vi "Periodic Tasks.vi"(8 "error in":errorcluster) -> ()   [LabVIEW 2013]
doc: "This VI runs in parallel to other tasks. It can contain as many user-defined periodic loops as you need. These can carry out PID or other sorts of timed response."
uses:
  <vilib>/Rock Robotics/SystemInterfaces/Utilities/FPGA_UtilitiesLED Source.ctl
  <vilib>/Rock Robotics/SystemInterfaces/Utilities/FPGA_UtilitiesLED State.ctl
  <vilib>/Rock Robotics/WPI/DriverStation/DriverStationLCD/WPI_DriverStationLCDLCDLine.ctl
  Robot Global Data.vi
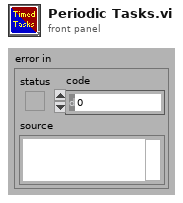
[diagram p1: front panel]
types:
  T1 = typedef "WPI_DigitalInputDevRef.ctl" = cluster{"DevStatus":errorcluster, "DIO Channel":T2, "Digital Module":T3}
  T2 = typedef "FPGA_DIOChannel.ctl" = enum8{"DIO 1", "DIO 2", "DIO 3", "DIO 4", "DIO 5", "DIO 6", "DIO 7", "DIO 8", "DIO 9", "DIO 10", "DIO 11", "DIO 12", "DIO 13", "DIO 14", "Invalid"}
  T3 = typedef "FPGA_TypedefDigitalModule.ctl" = enum16{"Digital Module 1", "Digital Module 2"}
  T4 = typedef "WPI_AnalogChannelDevRef.ctl" = cluster{"DevStatus":errorcluster, "Analog Module":T5, "Analog Channel":T6}
  T5 = typedef "FPGA_TypedefAnalogModule.ctl" = enum16{"Analog Module 1", "Analog Module 2"}
  T6 = typedef "FPGA_AIChannel.ctl" = enum8{"AI 1", "AI 2", "AI 3", "AI 4", "AI 5", "AI 6", "AI 7", "AI 8", "Invalid"}
  T7 = typedef "WPI_EncoderDevRef.ctl" = cluster{"DevStatus":errorcluster, "EncoderIndex":T8, "CounterIndex":T9, "DistancePerCount":dbl, "Decoding Type":T10}
  T8 = typedef "FPGA_EncoderIdx.ctl" = enum8{"Enc 0", "Enc 1", "Enc 2", "Enc 3", "Invalid"}
  T9 = typedef "FPGA_CounterCtrSystemIndex.ctl" = enum8{"Ctr 0", "Ctr 1", "Ctr 2", "Ctr 3", "Ctr 4", "Ctr 5", "Ctr 6", "Ctr 7", "Invalid"}
  T10 = typedef "WPI_EncoderType.ctl" = enum16{"1x", "2x", "4x"}
  T11 = cluster{"Winch Desired Location":dbl, "Winch Desired Location 2":dbl, "Winch Desired Location 3":dbl}
  T12 = typedef "FPGA_UtilitiesLED State.ctl" = enum16{"Off", "On", "Toggle"}
  T13 = typedef "FPGA_UtilitiesLED Source.ctl" = enum16{"User LED", "FPGA LED"}
  T14 = typedef "WPI_DriverStationLCDLCDLine.ctl" = enum16{"Main - Line 1", "User - Line 2", "User - Line 3", "User - Line 4", "User - Line 5", "User - Line 6"}
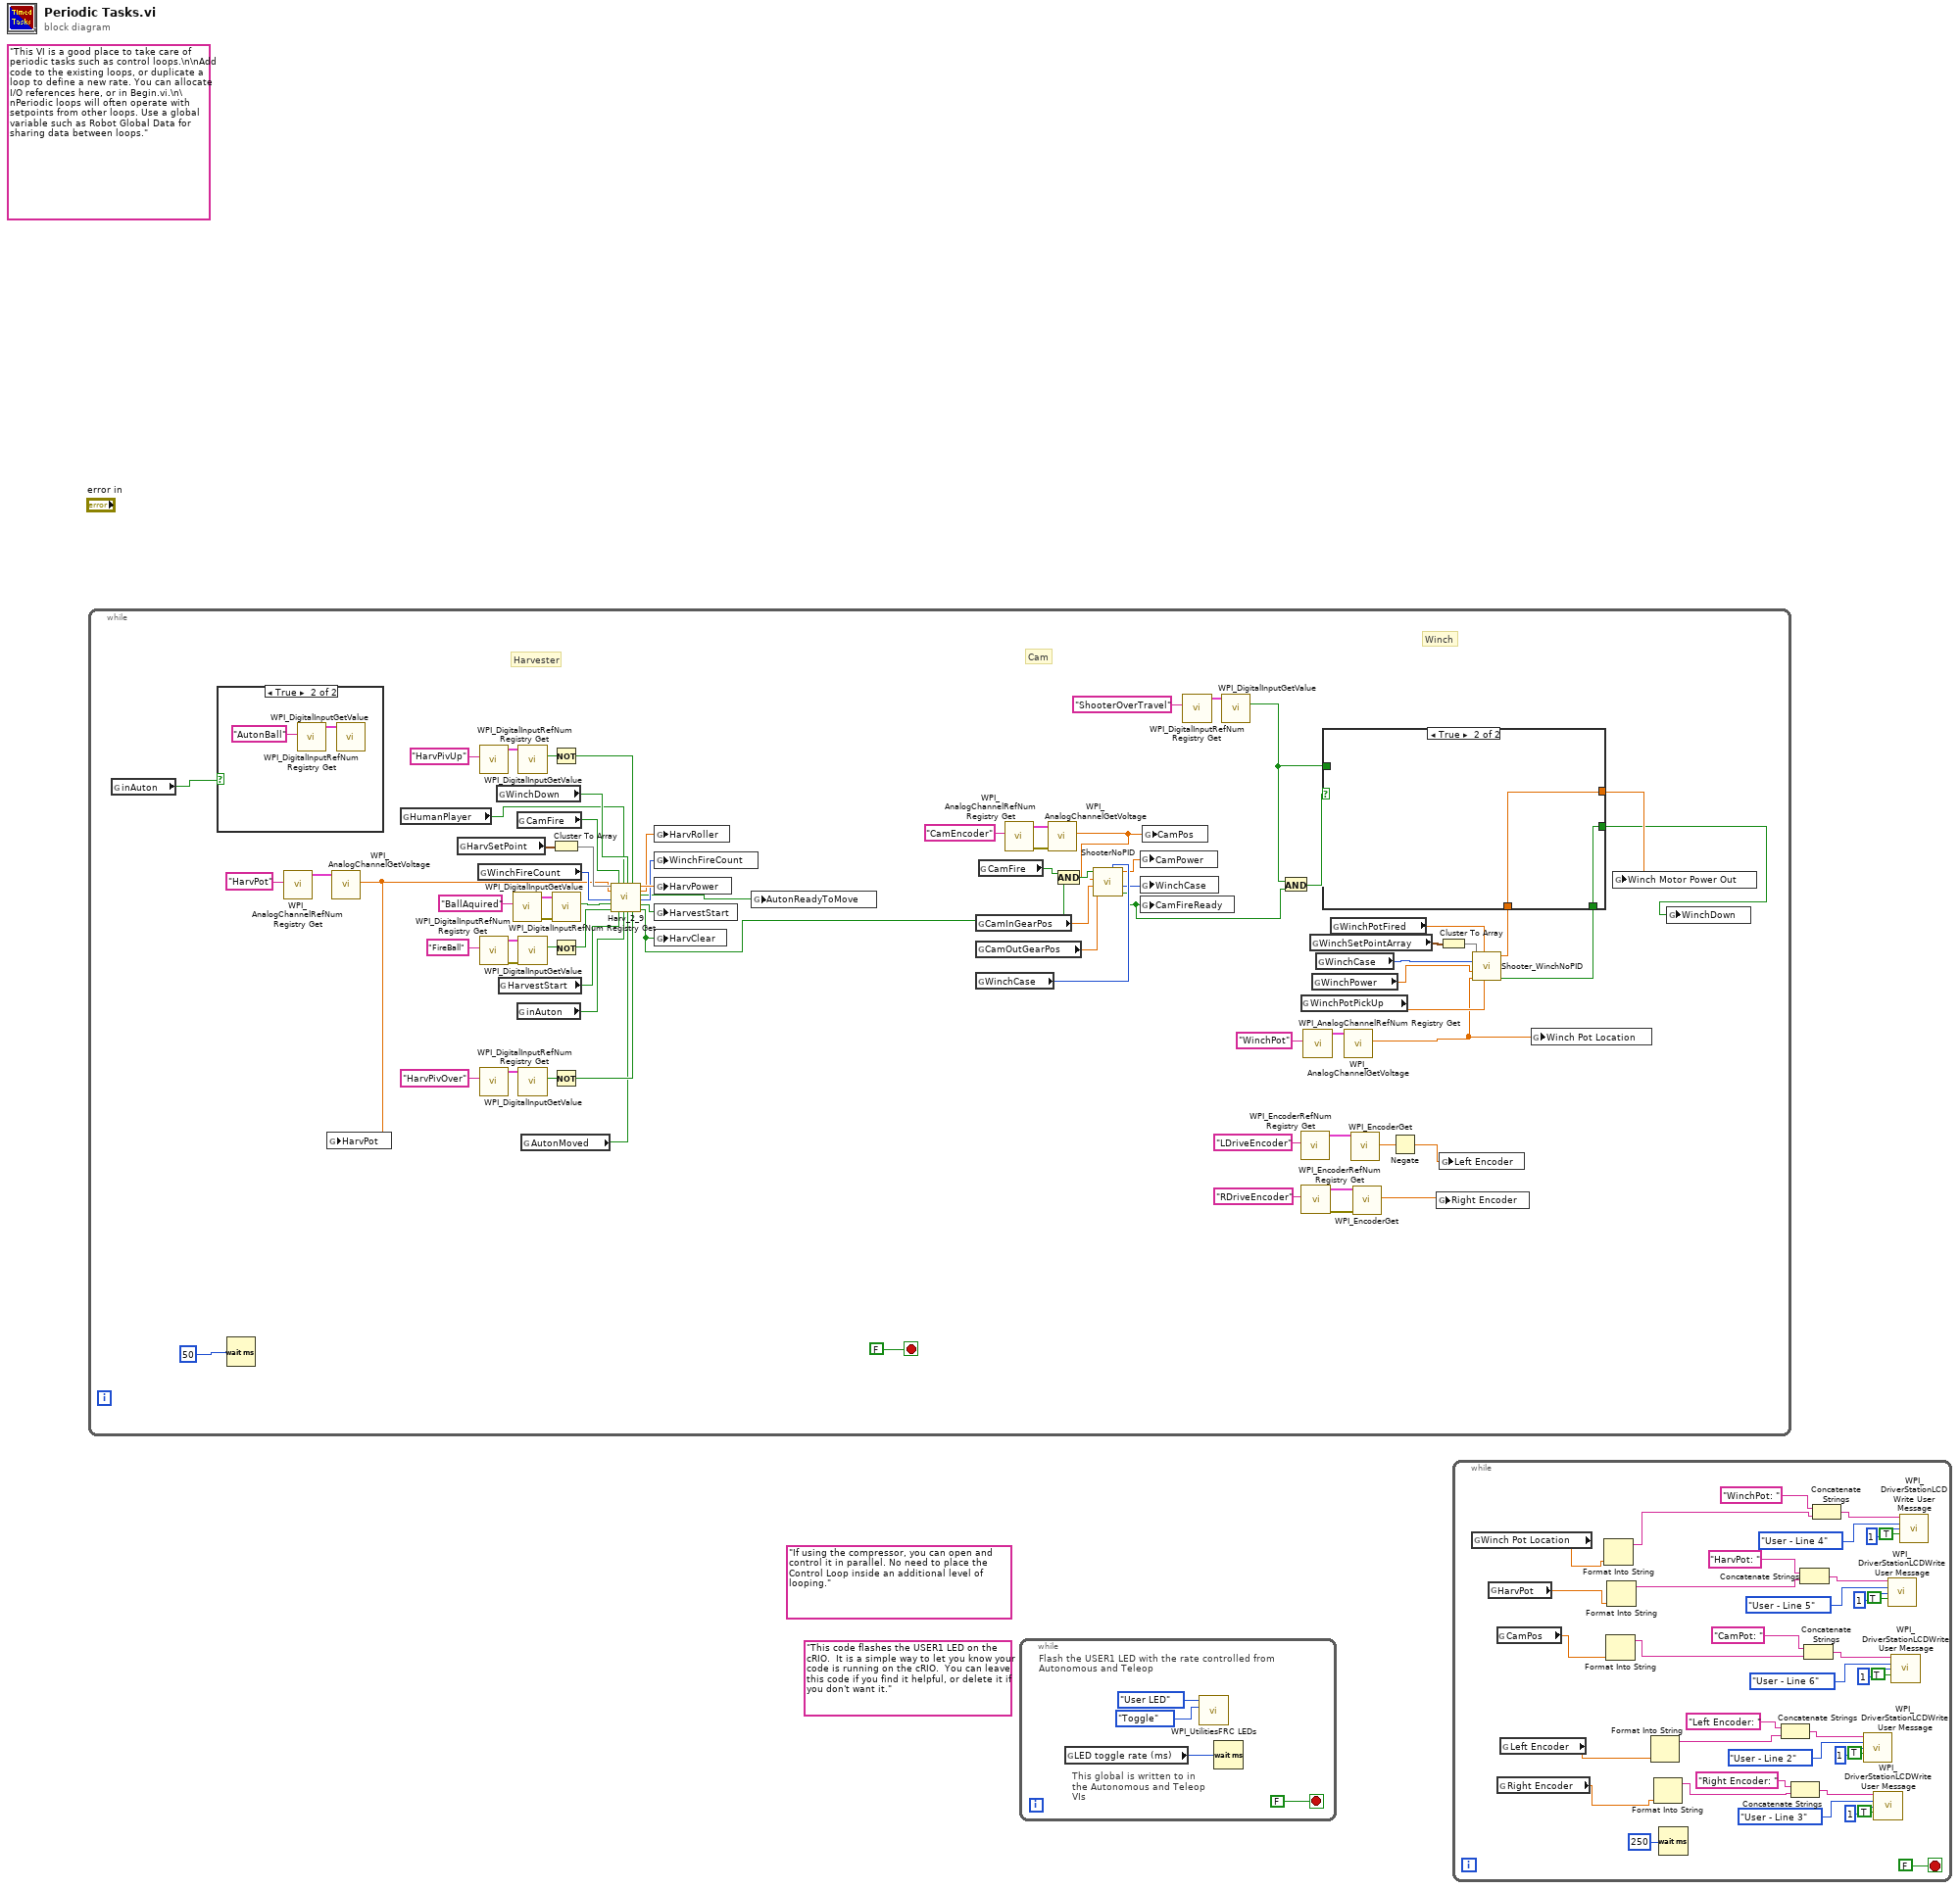
[diagram p0: block diagram]
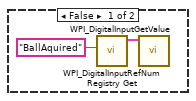
[diagram p2: hidden frame]
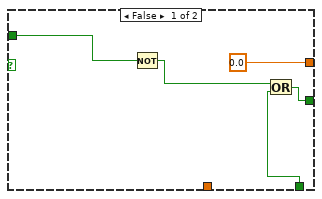
[diagram p3: hidden frame]
diagram:
  (unwired) "If using the compressor, you can open and control it in parallel. No need to place the Control Loop inside an additional level of looping."
  (unwired) "This code flashes the USER1 LED on the cRIO.  It is a simple way to let you know your code is running on the cRIO.  You can leave this code if you find it helpful, or delete it if you don't want it."
  (unwired) "This VI is a good place to take care of periodic tasks such as control loops.\n\nAdd code to the existing loops, or duplicate a loop to define a new rate. You can allocate I/O references here, or in Begin.vi.\n\nPeriodic loops will often operate with setpoints from other loops. Use a global variable such as Robot Global Data for sharing data between loops."
  n1 = while {
    stop <- FALSE stop-if-true
    # "Winch"
    # "Cam"
    # "Harvester"
    n2 = global read "Robot Global Data.vi" "inAuton"() -> (w1:bool)
    n3 = case shown="True" w1 {
      frame False {
        n4 = call <vilib>:"WPI_DigitalInputRefNum Registry Get.vi"("refnum name"="BallAquired") -> ("DigitalInputDevRef"=w77:T1)  [unwired: 9 in, 1 out]
        n5 = call <vilib>:"WPI_DigitalInputGetValue.vi"("DigitalInputDevRef"=w77) -> ()  [unwired: 8 in, 3 out]
      }
      frame True {
        n6 = call <vilib>:"WPI_DigitalInputRefNum Registry Get.vi"("refnum name"="AutonBall") -> ("DigitalInputDevRef"=w79:T1)  [unwired: 9 in, 1 out]
        n7 = call <vilib>:"WPI_DigitalInputGetValue.vi"("DigitalInputDevRef"=w79) -> ()  [unwired: 8 in, 3 out]
      }
    }
    n8 = Wait (ms)(milliseconds to wait=u32 50) -> ()  [unwired: 1 out]
    n9 = call <vilib>:"WPI_AnalogChannelRefNum Registry Get.vi"("refnum name"="HarvPot") -> ("AIDeviceRef"=w74:T4)  [unwired: 9 in, 1 out]
    n10 = call <vilib>:"WPI_AnalogChannelGetVoltage.vi"("AIDeviceRef"=w74) -> ("Voltage"=w13:dbl)  [unwired: 8 in, 2 out]
    n11 = global write "Robot Global Data.vi" "HarvPot"(w13) -> ()
    n12 = global read "Robot Global Data.vi" "HumanPlayer"() -> (w4:bool)
    n13 = global read "Robot Global Data.vi" "HarvSetPoint"() -> (w41:cluster{"Out":dbl, "In":dbl, "Clear":dbl})
    n14 = global read "Robot Global Data.vi" "WinchFireCount"() -> (w16:i32)
    n15 = call <vilib>:"WPI_DigitalInputRefNum Registry Get.vi"("refnum name"="HarvPivUp") -> ("DigitalInputDevRef"=w58:T1)  [unwired: 9 in, 1 out]
    n16 = call <vilib>:"WPI_DigitalInputRefNum Registry Get.vi"("refnum name"="FireBall") -> ("error out"=w47:errorcluster, "DigitalInputDevRef"=w48:T1)  [unwired: 9 in]
    n17 = call <vilib>:"WPI_DigitalInputRefNum Registry Get.vi"("refnum name"="HarvPivOver") -> ("DigitalInputDevRef"=w66:T1)  [unwired: 9 in, 1 out]
    n18 = global read "Robot Global Data.vi" "WinchDown"() -> (w34:bool)
    n19 = global read "Robot Global Data.vi" "HarvestStart"() -> (w45:bool)
    n20 = call <vilib>:"WPI_DigitalInputRefNum Registry Get.vi"("refnum name"="BallAquired") -> ("error out"=w54:errorcluster, "DigitalInputDevRef"=w53:T1)  [unwired: 9 in]
    n21 = global read "Robot Global Data.vi" "CamFire"() -> (w46:bool)
    n22 = global read "Robot Global Data.vi" "inAuton"() -> (w18:bool)
    n23 = call <vilib>:"WPI_DigitalInputGetValue.vi"("DigitalInputDevRef"=w58) -> ("Value"=w37:bool)  [unwired: 8 in, 2 out]
    n24 = call <vilib>:"WPI_DigitalInputGetValue.vi"("error in (no error)"=w47, "DigitalInputDevRef"=w48) -> ("Value"=w44:bool)  [unwired: 7 in, 2 out]
    n25 = call <vilib>:"WPI_DigitalInputGetValue.vi"("DigitalInputDevRef"=w66) -> ("Value"=w39:bool)  [unwired: 8 in, 2 out]
    n26 = global read "Robot Global Data.vi" "AutonMoved"() -> (w3:bool)
    n27 = Not(x=w37) -> (.not. x?=w36:bool)
    n28 = Cluster To Array(cluster=w41) -> (array=w40:dbl[])
    n29 = call <vilib>:"WPI_DigitalInputGetValue.vi"("error in (no error)"=w54, "DigitalInputDevRef"=w53) -> ("Value"=w43:bool)  [unwired: 7 in, 2 out]
    n30 = Not(x=w44) -> (.not. x?=w42:bool)
    n31 = Not(x=w39) -> (.not. x?=w38:bool)
    n32 = call "Harv_2_9.vi"("HarvSetpoints"=w40, "HarvPot"=w13, "Count"=w16, "BallAcquired"=w43, "FireBallSen"=w42, "Fire"=w46, "Harvest"=w45, "HPButton"=w4, "inAuton?"=w18, "WinchDown"=w34, "AutonMoved"=w3, "HarvPivUP"=w36, "HarvPivPickupLim"=w38) -> ("HarvPower"=w51:dbl, "HarvRoller"=w50:dbl, "AutonReadyToMove"=w2:bool, "CountOut"=w15:i32, "HarvStart"=w35:bool, "HarvCleared"=w8:bool)  [unwired: 1 in]
    n33 = global write "Robot Global Data.vi" "HarvRoller"(w50) -> ()
    n34 = global write "Robot Global Data.vi" "WinchFireCount"(w15) -> ()
    n35 = global write "Robot Global Data.vi" "HarvPower"(w51) -> ()
    n36 = global write "Robot Global Data.vi" "HarvestStart"(w35) -> ()
    n37 = global write "Robot Global Data.vi" "HarvClear"(w8) -> ()
    n38 = global write "Robot Global Data.vi" "AutonReadyToMove"(w2) -> ()
    n39 = global read "Robot Global Data.vi" "CamInGearPos"() -> (w23:dbl)
    n40 = global read "Robot Global Data.vi" "CamOutGearPos"() -> (w22:dbl)
    n41 = global read "Robot Global Data.vi" "WinchCase"() -> (w24:i32)
    n42 = global read "Robot Global Data.vi" "CamFire"() -> (w60:bool)
    n43 = call <vilib>:"WPI_AnalogChannelRefNum Registry Get.vi"("refnum name"="CamEncoder") -> ("error out"=w62:errorcluster, "AIDeviceRef"=w61:T4)  [unwired: 9 in]
    n44 = call <vilib>:"WPI_AnalogChannelGetVoltage.vi"("error in (no error)"=w62, "AIDeviceRef"=w61) -> ("Voltage"=w12:dbl)  [unwired: 7 in, 2 out]
    n45 = And(x=w60, y=w8) -> (x .and. y?=w25:bool)
    n46 = call "ShooterNoPID.vi"("WinchCaseIn"=w24, "InGearPosLow"=w22, "InGearPosHigh"=w23, "Pot"=w12, "Fire"=w25) -> ("There?"=w19:bool, "WinchCase"=w20:i32, "Power"=w21:dbl)  [unwired: 4 in]
    n47 = global write "Robot Global Data.vi" "CamPower"(w21) -> ()
    n48 = global write "Robot Global Data.vi" "WinchCase"(w20) -> ()
    n49 = global write "Robot Global Data.vi" "CamFireReady"(w19) -> ()
    n50 = global write "Robot Global Data.vi" "CamPos"(w12) -> ()
    n51 = call <vilib>:"WPI_DigitalInputRefNum Registry Get.vi"("refnum name"="ShooterOverTravel") -> ("DigitalInputDevRef"=w57:T1)  [unwired: 9 in, 1 out]
    n52 = call <vilib>:"WPI_DigitalInputGetValue.vi"("DigitalInputDevRef"=w57) -> ("Value"=w33:bool)  [unwired: 8 in, 2 out]
    n53 = And(x=w33, y=w19) -> (x .and. y?=w55:bool)
    n54 = global read "Robot Global Data.vi" "WinchPotPickUp"() -> (w17:dbl)
    n55 = call <vilib>:"WPI_EncoderRefNum Registry Get.vi"("refnum name"="LDriveEncoder") -> ("EncoderDevRef"=w68:T7)  [unwired: 9 in, 1 out]
    n56 = call <vilib>:"WPI_EncoderRefNum Registry Get.vi"("refnum name"="RDriveEncoder") -> ("error out"=w11:errorcluster, "EncoderDevRef"=w10:T7)  [unwired: 9 in]
    n57 = call <vilib>:"WPI_AnalogChannelRefNum Registry Get.vi"("refnum name"="WinchPot") -> ("AIDeviceRef"=w70:T4)  [unwired: 9 in, 1 out]
    n58 = global read "Robot Global Data.vi" "WinchSetPointArray"() -> (w30:T11)
    n59 = global read "Robot Global Data.vi" "WinchPower"() -> (w32:dbl)
    n60 = global read "Robot Global Data.vi" "WinchCase"() -> (w29:i32)
    n61 = global read "Robot Global Data.vi" "WinchPotFired"() -> (w5:dbl)
    n62 = call <vilib>:"WPI_AnalogChannelGetVoltage.vi"("AIDeviceRef"=w70) -> ("Voltage"=w14:dbl)  [unwired: 8 in, 2 out]
    n63 = call <vilib>:"WPI_EncoderGet.vi"("EncoderDevRef"=w68) -> ("Distance"=w7:dbl)  [unwired: 5 in, 5 out]
    n64 = call <vilib>:"WPI_EncoderGet.vi"("error in (no error)"=w11, "EncoderDevRef"=w10) -> ("Distance"=w9:dbl)  [unwired: 4 in, 5 out]
    n65 = Negate(x=w7) -> (-x=w6:dbl)
    n66 = global write "Robot Global Data.vi" "Right Encoder"(w9) -> ()
    n67 = Cluster To Array(cluster=w30) -> (array=w31:dbl[])
    n68 = global write "Robot Global Data.vi" "Left Encoder"(w6) -> ()
    n69 = call "Shooter_WinchNoPID.vi"("PickStartPos"=w17, "WinchFiredPos"=w5, "Winch Pot Location"=w14, "WinchPower"=w32, "selectedCase"=w29, "SetPointArray"=w31) -> ("isThere?"=w27:bool, "Winch Motor Power Out"=w26:dbl)  [unwired: 4 in]
    n70 = case shown="True" w55 {
      tunnel: [0.0 ("Winch Motor Power Out") w85] -> w64
      tunnel: [w83 w86] -> w28
      tunnel: w33 -> [w82 _]
      tunnel: w27 -> [w80 w86]
      tunnel: w26 -> [_ w85]
      frame False {
        n71 = Not(x=w82) -> (.not. x?=w81:bool)
        n72 = Or(x=w81, y=w80) -> (x .or. y?=w83:bool)
      }
      frame True {
      }
    }
    n73 = global write "Robot Global Data.vi" "Winch Pot Location"(w14) -> ()
    n74 = global write "Robot Global Data.vi" "Winch Motor Power Out"(w64) -> ()
    n75 = global write "Robot Global Data.vi" "WinchDown"(w28) -> ()
  }
  n76 = while {
    stop <- FALSE stop-if-true
    # "This global is written to in the Autonomous and Teleop VIs"
    # "Flash the USER1 LED with the rate controlled from Autonomous and Teleop"
    n77 = global read "Robot Global Data.vi" "LED toggle rate (ms)"() -> (w87:u32)
    n78 = call <vilib>:"WPI_UtilitiesFRC LEDs.vi"("State"=FPGA_UtilitiesLED_State."Toggle", "LED Type"=FPGA_UtilitiesLED_Source."User LED") -> ()  [unwired: 1 in, 9 out]
    n79 = Wait (ms)(milliseconds to wait=w87) -> ()  [unwired: 1 out]
  }
  n80 = while {
    stop <- FALSE stop-if-true
    n81 = global read "Robot Global Data.vi" "Winch Pot Location"() -> (w96:dbl)
    n82 = global read "Robot Global Data.vi" "HarvPot"() -> (w95:dbl)
    n83 = global read "Robot Global Data.vi" "CamPos"() -> (w97:dbl)
    n84 = global read "Robot Global Data.vi" "Right Encoder"() -> (w93:dbl)
    n85 = global read "Robot Global Data.vi" "Left Encoder"() -> (w94:dbl)
    n86 = Format Into String(w96) -> (resulting string=w113:string)  [unwired: 3 in, 1 out]
    n87 = Format Into String(w97) -> (resulting string=w98:string)  [unwired: 3 in, 1 out]
    n88 = Format Into String(w95) -> (resulting string=w107:string)  [unwired: 3 in, 1 out]
    n89 = Format Into String(w94) -> (resulting string=w105:string)  [unwired: 3 in, 1 out]
    n90 = Format Into String(w93) -> (resulting string=w104:string)  [unwired: 3 in, 1 out]
    n91 = Wait (ms)(milliseconds to wait=u32 250) -> ()  [unwired: 1 out]
    n92 = Concatenate Strings("Left Encoder: ", w105) -> (w123:string)
    n93 = Concatenate Strings("Right Encoder: ", w104) -> (w122:string)
    n94 = Concatenate Strings("HarvPot: ", w107) -> (w108:string)
    n95 = Concatenate Strings("CamPot: ", w98) -> (w103:string)
    n96 = Concatenate Strings("WinchPot: ", w113) -> (w118:string)
    n97 = call <vilib>:"WPI_DriverStationLCDWrite User Message.vi"("line text"=w123, "line"=WPI_DriverStationLCDLCDLine."User - Line 2", "starting column"=i8 1, "clear line before write (T)"=TRUE) -> ()  [unwired: 1 in, 11 out]
    n98 = call <vilib>:"WPI_DriverStationLCDWrite User Message.vi"("line text"=w122, "line"=WPI_DriverStationLCDLCDLine."User - Line 3", "starting column"=i8 1, "clear line before write (T)"=TRUE) -> ()  [unwired: 1 in, 11 out]
    n99 = call <vilib>:"WPI_DriverStationLCDWrite User Message.vi"("line text"=w108, "line"=WPI_DriverStationLCDLCDLine."User - Line 5", "starting column"=i8 1, "clear line before write (T)"=TRUE) -> ()  [unwired: 1 in, 11 out]
    n100 = call <vilib>:"WPI_DriverStationLCDWrite User Message.vi"("line text"=w103, "line"=WPI_DriverStationLCDLCDLine."User - Line 6", "starting column"=i8 1, "clear line before write (T)"=TRUE) -> ()  [unwired: 1 in, 11 out]
    n101 = call <vilib>:"WPI_DriverStationLCDWrite User Message.vi"("line text"=w118, "line"=WPI_DriverStationLCDLCDLine."User - Line 4", "starting column"=i8 1, "clear line before write (T)"=TRUE) -> ()  [unwired: 1 in, 11 out]
  }
